vi "_Electronic On.vi"   [LabVIEW 2012]
uses:
  <vilib>/eio/EIONode/EIONode.xnode
  <vilib>/rvi/DataTransferAndStorage/Container/XNode/niFpgaContainer.xnode
  <vilib>/rvi/Memory/Memory_Emulation/nirvimemoryEmulation.vi
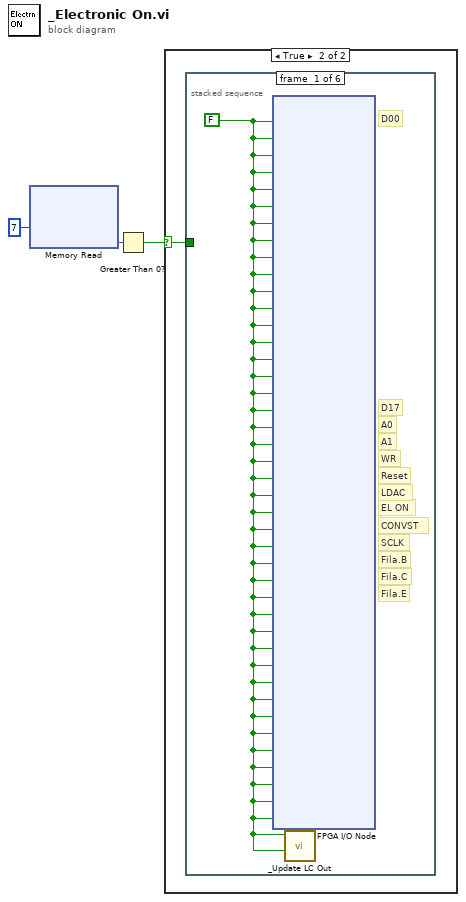
[diagram p0: block diagram]
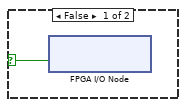
[diagram p2: hidden frame]
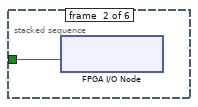
[diagram p3: hidden frame]
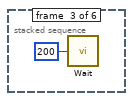
[diagram p4: hidden frame]
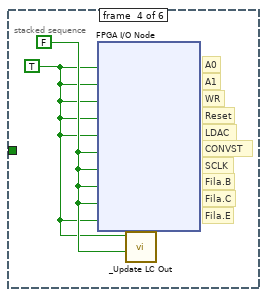
[diagram p5: hidden frame]
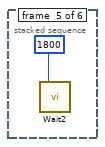
[diagram p6: hidden frame]
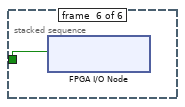
[diagram p7: hidden frame]
diagram:
  n1 = xnode ("Memory Read")("Address"=u8 7) -> ("Data"=w3:i16)  [unwired: 1 in, 1 out]
  n2 = Greater Than 0?(x=w3) -> (x > 0?=w1:bool)
  n3 = case shown="True" w1 {
    selector: w1 -> [w4 w5]
    frame False {
      n4 = xnode "FPGA I/O Node"("Port2/DIO9"=w4) -> ()  [unwired: 1 in, 1 out]
    }
    frame True {
      n5 = stacked-sequence {
        tunnel: w5 -> [_ w7 _ _ _ w12]
        frame #0 {
          w6 = FALSE ("Port4/DIO8")
          # "Fila.E"
          # "Fila.C"
          # "Fila.B"
          # "SCLK"
          # "CONVST"
          # "EL ON"
          # "LDAC"
          # "WR"
          # "A1"
          # "A0"
          # "Reset"
          # "D17"
          # "D00"
          n6 = xnode "FPGA I/O Node"("Port4/DIO8"=w6, "Port4/DIO7"=w6, "Port4/DIO6"=w6, "Port4/DIO5"=w6, "Port4/DIO4"=w6, "Port4/DIO3"=w6, "Port4/DIO2"=w6, "Port4/DIO1"=w6, "Port4/DIO0"=w6, "Port3/DIO8"=w6, "Port3/DIO7"=w6, "Port3/DIO6"=w6, "Port3/DIO5"=w6, "Port3/DIO4"=w6, "Port3/DIO3"=w6, "Port3/DIO2"=w6, "Port3/DIO1"=w6, "Port3/DIO0"=w6, "Port7/DIO1"=w6, "Port7/DIO0"=w6, "Port7/DIO3"=w6, "Port1/DIO4"=w6, "Port7/DIO2"=w6, "Port2/DIO9"=w6, "Port6/DIO4"=w6, "Port6/DIO5"=w6, "Port2/DIO5"=w6, "Port2/DIO6"=w6, "Port2/DIO7"=w6, "Port0/DIO8"=w6, "Port1/DIO0"=w6, "Port1/DIO1"=w6, "Port1/DIO2"=w6, "Port1/DIO3"=w6, "Port1/DIO5"=w6, "Port1/DIO6"=w6, "Port1/DIO7"=w6, "Port1/DIO8"=w6, "Port2/DIO0"=w6, "Port2/DIO1"=w6, "Port2/DIO2"=w6, "Port2/DIO3"=w6) -> ()  [unwired: 42 in, 42 out]
          n7 = call "_Update LC Out.vi"("LC Stop"=w6, "LC Hold"=w6) -> ()  [unwired: 6 out]
        }
        frame #1 {
          n8 = xnode "FPGA I/O Node"("Port2/DIO9"=w7) -> ()  [unwired: 1 in, 1 out]
        }
        frame #2 {
          n9 = call "Wait"("Count(mSec)"=u8 200) -> ()  [unwired: 1 out]
        }
        frame #3 {
          w9 = TRUE
          w10 = FALSE ("Port4/DIO8")
          # "Fila.E"
          # "Fila.C"
          # "Fila.B"
          # "SCLK"
          # "CONVST"
          # "LDAC"
          # "WR"
          # "A1"
          # "A0"
          # "Reset"
          n10 = xnode "FPGA I/O Node"("Port7/DIO1"=w9, "Port7/DIO0"=w9, "Port7/DIO3"=w9, "Port1/DIO4"=w9, "Port7/DIO2"=w9, "Port6/DIO4"=w10, "Port6/DIO5"=w10, "Port2/DIO5"=w10, "Port2/DIO6"=w10, "Port2/DIO7"=w9) -> ()  [unwired: 10 in, 10 out]
          n11 = call "_Update LC Out.vi"("LC Stop"=w10, "LC Hold"=w9) -> ()  [unwired: 6 out]
        }
        frame #4 {
          n12 = call "Wait2"("Count(mSec)"=u16 1800) -> ()  [unwired: 1 out]
        }
        frame #5 {
          n13 = xnode "FPGA I/O Node"("Port6/DIO4"=w12) -> ()  [unwired: 1 in, 1 out]
        }
      }
    }
  }
